vi "CalcMotorCurrent.vi"(8 "Reference Voltage (12)":dbl=12.0, 9 "Motor Characteristics":T1, 10 "Motor Torque":dbl, 11 "Motor Voltage":dbl) -> (3 "Motor Current":dbl)   [LabVIEW 2014]
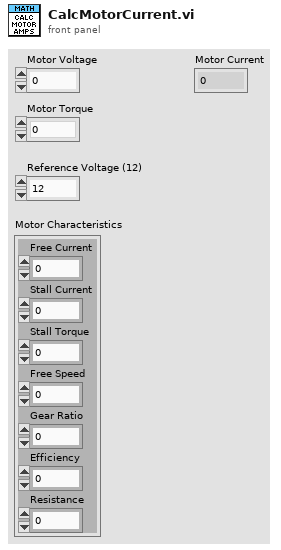
[diagram p1: front panel]
types:
  T1 = cluster{"Free Current":dbl, "Stall Current":dbl, "Stall Torque":dbl, "Free Speed":dbl, "Gear Ratio":dbl, "Efficiency":dbl, "Resistance":dbl}
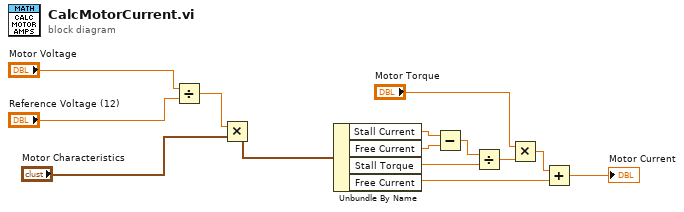
[diagram p0: block diagram]
diagram:
  n1 = Divide(x="Motor Voltage", y="Reference Voltage (12)") -> (x/y=w12:dbl)
  n2 = Multiply(x=w12, y="Motor Characteristics") -> (x*y=w10:T1)
  n3 = Unbundle By Name(w10) -> ("Stall Current"=w9:dbl, "Free Current"=w8:dbl, "Stall Torque"=w6:dbl, "Free Current"=w2:dbl)
  n4 = Subtract(x=w9, y=w8) -> (x-y=w7:dbl)
  n5 = Divide(x=w7, y=w6) -> (x/y=w5:dbl)
  n6 = Multiply(x="Motor Torque", y=w5) -> (x*y=w3:dbl)
  n7 = Add(x=w3, y=w2) -> (x+y=→"Motor Current":dbl)
